vi "UE9 PWM Output and 32-bit Frequency Input.vi"(8 "error in":errorcluster, 9 "PWM16 Duty Cycle [%]":dbl=50.0 format="%.1f") -> (2 "Period Input [s]":dbl format="%.6f")   [LabVIEW 2021]
panel:
  out "Frequency Input [Hz]":dbl format="%.2f"
  out "Timer Value Array":u16[](array[numeric])
  in  "stop":bool
  in  "FirstFound":bool=TRUE
  in  "Address":string="1"
  in  "ConnectionType":u16(ring) items=["LJ_ctUSB", "LJ_ctETHERNET"]
  out "Error Message":string
  # "Demonstrates 1 32-bit period measurement (FIO0) with 1 PWM16 output (FIO1).\n\nFor testing, wire FIO0 to FIO1.  The default output on FIO1 is 183 Hz."
  # "This VI allows the duty cycle to\nbe changed while the VI is running."
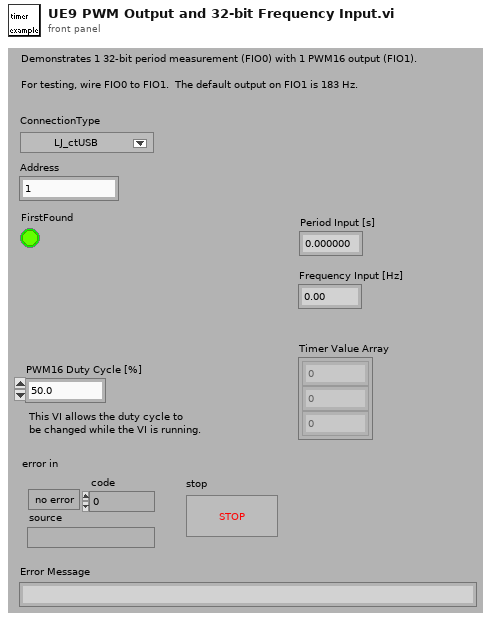
[diagram p1: front panel]
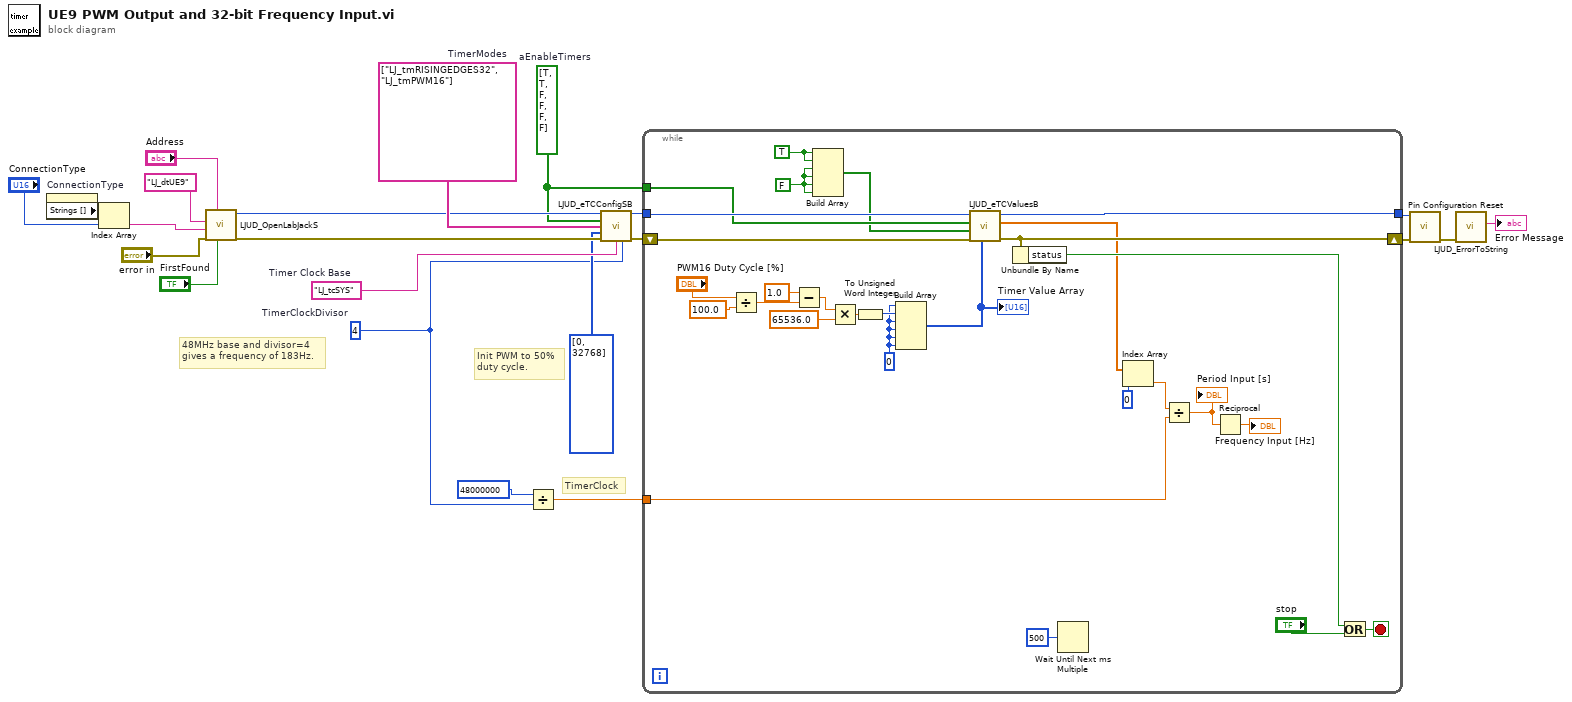
[diagram p0: block diagram]
diagram:
  w2 = 4  # TimerClockDivisor
  w6 = "LJ_tcSYS"  # Timer Clock Base
  w5 = bool[] [TRUE, TRUE, FALSE, FALSE, FALSE, FALSE]  # aEnableTimers
  w9 = string[] ["LJ_tmRISINGEDGES32", "LJ_tmPWM16"]  # TimerModes
  # "TimerClock"
  # "48MHz base and divisor=4\ngives a frequency of 183Hz."
  # "Init PWM to 50%\nduty cycle."
  n1 = property on="ConnectionType" class="Ring (strict)"() -> ("Strings []"=w17:string[])  [unwired: 2 in, 2 out]
  n2 = Index Array(array=w17, index="ConnectionType") -> (element=w15:string)
  n3 = call "LJUD_OpenLabJackS.vi"("FirstFound"="FirstFound", "Address"="Address", "error in"="error in", "ConnectionType"=w15, "DeviceType"="LJ_dtUE9") -> ("error out"=w7:errorcluster, "Handle"=w8:i32)  [unwired: 4 in, 1 out]
  n4 = Divide(x=u32 48000000, y=w2) -> (x/y=w1:dbl)
  n5 = call "LJUD_eTCConfigSB.vi"("Handle In"=w8, "aEnableTimers"=w5, "aTimerModes"=w9, "aTimerValues"=u16[] [0, 32768] ("TimerValues"), "error in"=w7, "TimerClockBase"=w6, "TimerClockDivisor"=w2) -> ("Handle Out"=w14:i32, "error out"=w13:errorcluster)  [unwired: 7 in]
  n6 = while {
    tunnel: w1 -> [w25]
    tunnel: w5 -> [w42]
    tunnel: [w46] -> w12
    tunnel: w14 -> [w49]
    shift-left: w13 -> [w50]
    shift-right: [w47] -> w11
    stop <- w48 stop-if-true
    w31 = TRUE ("Input Element")
    w30 = FALSE ("Input Element")
    w28 = u16 0 ("PWM Timer Value")
    n7 = Divide(x="PWM16 Duty Cycle [%]", y=100.0) -> (x/y=w37:dbl)
    n8 = Subtract(x=1.0, y=w37) -> (x-y=w35:dbl)
    n9 = Build Array(w31, w31, w30, w30, w30, w30) -> (w32:bool[])
    n10 = Multiply(x=w35, y=65536.0) -> (x*y=w34:dbl)
    n11 = To Unsigned Word Integer(number=w34) -> (unsigned 16bit integer=w29:u16)
    n12 = Build Array(w28, w29, w28, w28, w28, w28) -> (w27:u16[])
    "Timer Value Array" <- w27
    n13 = call "LJUD_eTCValuesB.vi"("aTimerValues Write"=w27, "error in"=w50, "aUpdateResetTimers"=w32, "aReadTimers"=w42, "Handle In"=w49) -> ("error out"=w47:errorcluster, "aTimerValues Read"=w40:dbl[], "Handle Out"=w46:i32)  [unwired: 3 in, 1 out]
    n14 = Unbundle By Name(w47) -> ("status"=w45:bool)
    n15 = Wait Until Next ms Multiple(millisecond multiple=u32 500) -> ()  [unwired: 1 out]
    n16 = Index Array(array=w40, index=0 ("Index")) -> (element=w26:dbl)
    n17 = Divide(x=w26, y=w25) -> (x/y=w24:dbl)
    "Period Input [s]" <- w24
    n18 = Reciprocal(x=w24) -> (1/x=→"Frequency Input [Hz]":dbl)
    n19 = Or(x=w45, y="stop") -> (x .or. y?=w48:bool)
  }
  n20 = call "Pin Configuration Reset.vi"("error in"=w11, "Handle In"=w12) -> ("error out"=w10:errorcluster)  [unwired: 8 in, 1 out]
  n21 = call "LJUD_ErrorToString.vi"("error in"=w10) -> ("String"=→"Error Message":string)  [unwired: 10 in]
